vi "Generate_WayPoints_Hopping.vi"(11 "Input Cluster":T2={"Scan Rate (um/s)"=15.0, "X Start"=15.0, "X End"=15.0, "Y Start"=15.0, "Y End"=15.0, " Z Start"=15.0, "HoppingDistance"=1.0, "V"=15.0, "Z End"=15.0, "Approach Rate Hopping (um/s)"=15.0, "Retract Rate (um/s)"=15.0, "V 2"=15.0, "Approach Rate (um/s)"=15.0, "RetractV (V "=15.0}) -> (0 "output cluster":T1)   [LabVIEW 2023]
uses:
  TypeDefs/WayPointCluster.ctl
  User_Vi/Settings.vi
panel:
  in  "WayPointCluster":T1
  out "Y  P":dbl
  out "X  P":dbl
  out "HoppingDistanceX":dbl
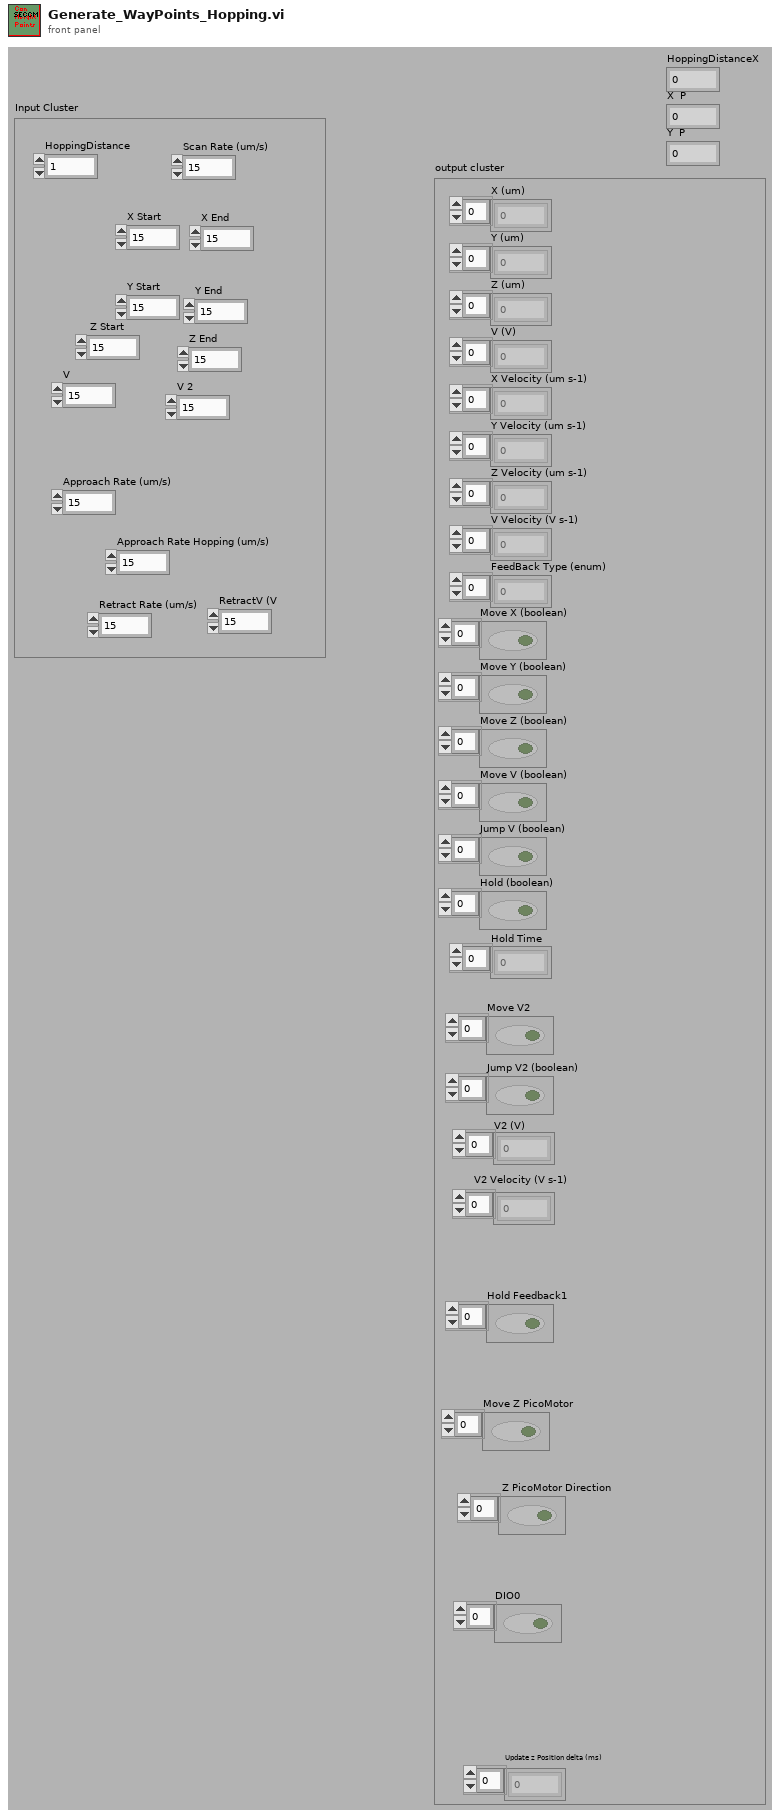
[diagram p1: front panel]
types:
  T1 = typedef "WayPointCluster.ctl" = cluster{"X (um)":dbl[], "Y (um)":dbl[], "Z (um)":dbl[], "V (V)":dbl[], "X Velocity (um s-1)":dbl[], "Y Velocity (um s-1)":dbl[], "Z Velocity (um s-1)":dbl[], "V Velocity (V s-1)":dbl[], "FeedBack Type (enum)":u16[], "Move X (boolean)":bool[], "Move Y (boolean)":bool[], "Move Z (boolean)":bool[], "Move V (boolean)":bool[], "Jump V (boolean)":bool[], "Hold (boolean)":bool[], "Hold Time":u32[], "V2 (V)":dbl[], "Move V2":bool[], "V2 Velocity (V s-1)":dbl[], "Jump V2 (boolean)":bool[], "Update z Position delta (ms)":i16[], "Hold Feedback1":bool[], "Move Z PicoMotor":bool[], " Z PicoMotor Direction":bool[], "DIO0":bool[]}
  T2 = cluster{"Scan Rate (um/s)":dbl, "X Start":dbl, "X End":dbl, "Y Start":dbl, "Y End":dbl, " Z Start":dbl, "HoppingDistance":dbl, "V":dbl, "Z End":dbl, "Approach Rate Hopping (um/s)":dbl, "Retract Rate (um/s)":dbl, "V 2":dbl, "Approach Rate (um/s)":dbl, "RetractV (V ":dbl}
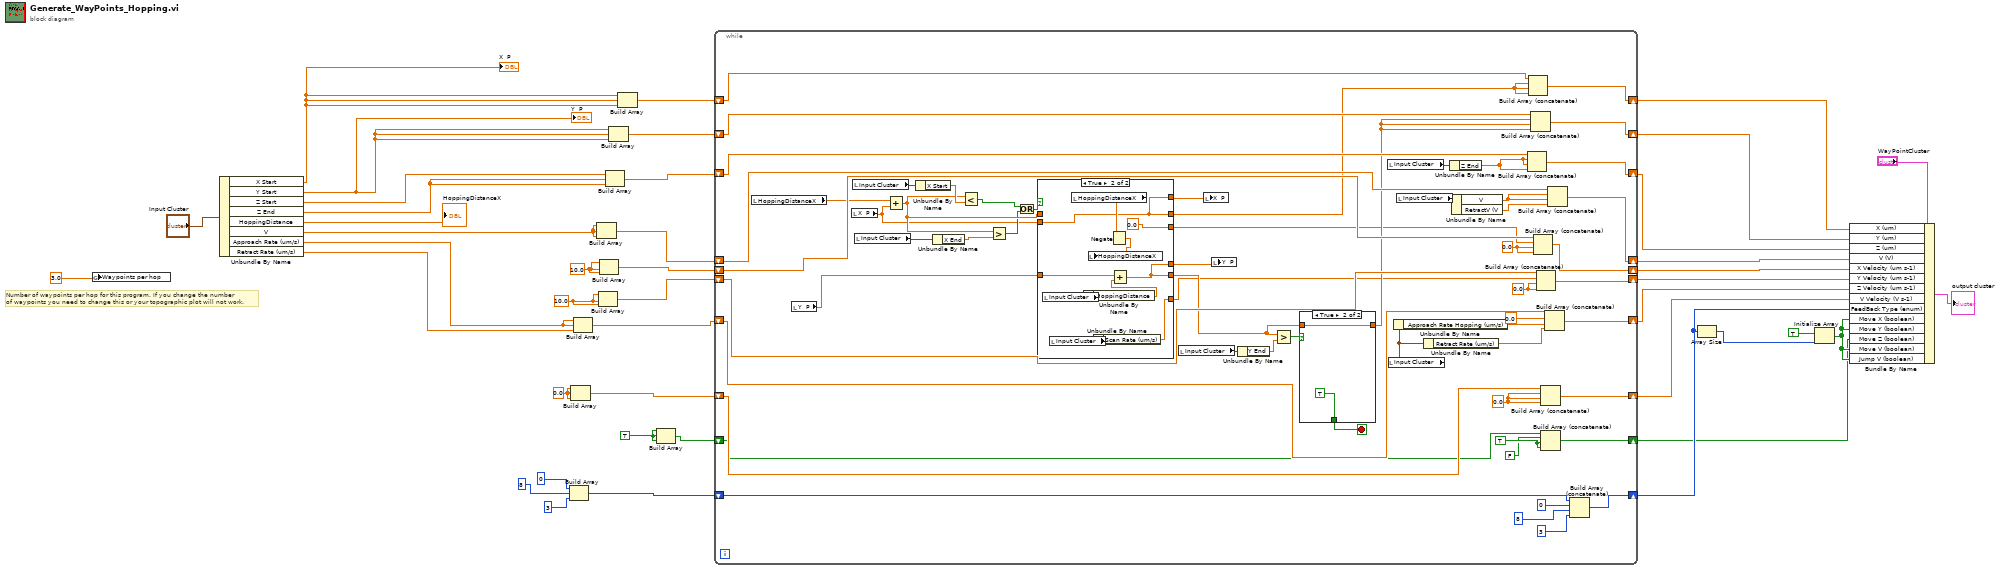
[diagram p0: block diagram]
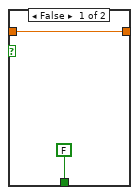
[diagram p2: hidden frame]
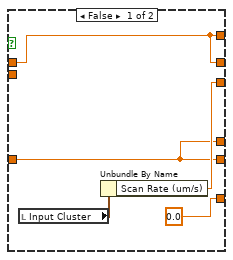
[diagram p3: hidden frame]
diagram:
  w2 = TRUE
  w12 = 10.0 ("element")
  w11 = 10.0 ("element")
  w9 = 0.0 ("element")
  # "Number of waypoints per hop for this program. If you change the number\nof waypoints you need to change this or your topographic plot will not work."
  n1 = global write "Settings.vi" "Waypoints per hop"(3.0) -> ()
  n2 = Unbundle By Name("Input Cluster") -> ("X Start"=w24:dbl, "Y Start"=w18:dbl, "Z Start"=w17:dbl, "Z End"=w14:dbl, "HoppingDistance"=→"HoppingDistanceX":dbl, "V"=w15:dbl, "Approach Rate (um/s)"=w10:dbl, "Retract Rate (um/s)"=w23:dbl)
  "X  P" <- w24
  "Y  P" <- w18
  n3 = Build Array(u16 0 ("element"), u16 8 ("element"), u16 3 ("element")) -> (w25:u16[])
  n4 = Build Array(w9, w9, w9) -> (w27:dbl[])
  n5 = Build Array(w10, w10, w23) -> (w29:dbl[])
  n6 = Build Array(w15, w15, w15) -> (w34:dbl[])
  n7 = Build Array(w11, w11, w11) -> (w31:dbl[])
  n8 = Build Array(w12, w12, w12) -> (w32:dbl[])
  n9 = Build Array(w17, w14, w14) -> (w36:dbl[])
  n10 = Build Array(w18, w18, w18) -> (w37:dbl[])
  n11 = Build Array(w24, w24, w24) -> (w39:dbl[])
  n12 = Build Array(w2, w2, w2) -> (w3:bool[])
  n13 = while {
    shift-right: [w98] -> w38
    shift-left: w39 -> [w99]
    shift-right: [w90] -> w19
    shift-left: w37 -> [w80]
    shift-right: [w89] -> w35
    shift-left: w36 -> [w97]
    shift-right: [w88] -> w33
    shift-left: w34 -> [w96]
    shift-right: [w87] -> w20
    shift-left: w32 -> [w95]
    shift-right: [w86] -> w30
    shift-left: w31 -> [w94]
    shift-right: [w85] -> w28
    shift-left: w29 -> [w93]
    shift-right: [w84] -> w26
    shift-left: w27 -> [w92]
    shift-right: [w83] -> w16
    shift-left: w25 -> [w91]
    shift-right: [w45] -> w4
    shift-left: w3 -> [w44]
    stop <- w70 stop-if-true
    w47 = TRUE
    w52 = 0.0 ("element")
    w53 = 0.0 ("element")
    w66 = 0.0 ("element")
    n14 = local read "HoppingDistanceX"() -> (w49:dbl)
    n15 = local read "Y  P"() -> (w64:dbl)
    n16 = local read "X  P"() -> (w50:dbl)
    n17 = local read "Input Cluster"() -> (w101:T2)
    n18 = local read "Input Cluster"() -> (w100:T2)
    n19 = Add(x=w49, y=w50) -> (x+y=w76:dbl)
    n20 = Unbundle By Name(w101) -> ("X Start"=w79:dbl)
    n21 = Unbundle By Name(w100) -> ("X End"=w77:dbl)
    n22 = Less?(x=w76, y=w79) -> (x < y?=w78:bool)
    n23 = Greater?(x=w76, y=w77) -> (0:w75:bool)
    n24 = Or(x=w78, y=w75) -> (x .or. y?=w74:bool)
    n25 = case shown="True" w74 {
      tunnel: w76 -> [w106 _]
      tunnel: [w106 w112] -> w63
      tunnel: w50 -> [_ w112]
      tunnel: w64 -> [w107 w113]
      tunnel: [w107 w111] -> w62
      tunnel: [w109 0.0] -> w54
      tunnel: [0.0 w114] -> w51
      tunnel: [w107 w111] -> w61
      tunnel: [w106 w112] -> w60
      frame False {
        n26 = local read "Input Cluster"() -> (w110:T2)
        n27 = Unbundle By Name(w110) -> ("Scan Rate (um/s)"=w109:dbl)
      }
      frame True {
        n28 = local read "Input Cluster"() -> (w118:T2)
        n29 = local read "Input Cluster"() -> (w116:T2)
        n30 = local read "HoppingDistanceX"() -> (w120:dbl)
        n31 = Unbundle By Name(w118) -> ("HoppingDistance"=w117:dbl)
        n32 = Unbundle By Name(w116) -> ("Scan Rate (um/s)"=w114:dbl)
        n33 = Negate(x=w120) -> (-x=w119:dbl)
        n34 = local write "HoppingDistanceX"(w119) -> ()
        n35 = Add(x=w113, y=w117) -> (x+y=w111:dbl)
      }
    }
    n36 = local read "Input Cluster"() -> (w73:T2)
    n37 = local write "X  P"(w60) -> ()
    n38 = local write "Y  P"(w61) -> ()
    n39 = Unbundle By Name(w73) -> ("Y End"=w72:dbl)
    n40 = Greater?(x=w62, y=w72) -> (0:w71:bool)
    n41 = case shown="True" w71 {
      tunnel: w62 -> [w103 w105]
      tunnel: [w103 w105] -> w69
      tunnel: [FALSE TRUE] -> w70
      frame False {
      }
      frame True {
      }
    }
    n42 = local read "Input Cluster"() -> (w82:T2)
    n43 = local read "Input Cluster"() -> (w65:T2)
    n44 = Unbundle By Name(w65) -> ("Approach Rate Hopping (um/s)"=w56:dbl)
    n45 = local read "Input Cluster"() -> (w81:T2)
    n46 = Unbundle By Name(w65) -> ("Retract Rate (um/s)"=w55:dbl)
    n47 = Unbundle By Name(w82) -> ("Z End"=w68:dbl)
    n48 = Unbundle By Name(w81) -> ("V"=w67:dbl, "RetractV (V"=w43:dbl)
    n49 = Build Array (concatenate)(w97, w68, w68, w68) -> (w89:dbl[])
    n50 = Build Array (concatenate)(w99, w63, w63, w63) -> (w98:dbl[])
    n51 = Build Array (concatenate)(w80, w69, w69, w69) -> (w90:dbl[])
    n52 = Build Array (concatenate)(w95, w54, w53, w53) -> (w87:dbl[])
    n53 = Build Array (concatenate)(w94, w51, w52, w52) -> (w86:dbl[])
    n54 = Build Array (concatenate)(w92, w66, w66, w66) -> (w84:dbl[])
    n55 = Build Array (concatenate)(w44, FALSE, w47, w47) -> (w45:bool[])
    n56 = Build Array (concatenate)(w93, 0.0 ("element"), w56, w55) -> (w85:dbl[])
    n57 = Build Array (concatenate)(w96, w67, w67, w43) -> (w88:dbl[])
    n58 = Build Array (concatenate)(w91, u16 0 ("element"), u16 8 ("element"), u16 3 ("element")) -> (w83:u16[])
  }
  n59 = Array Size(array=w16) -> (size(s)=w21:i32)
  n60 = Initialize Array(TRUE, w21) -> (w40:bool[])
  n61 = Bundle By Name(cluster="WayPointCluster", "X (um)"=w38, "Y (um)"=w19, "Z (um)"=w35, "V (V)"=w33, "X Velocity (um s-1)"=w20, "Y Velocity (um s-1)"=w30, "Z Velocity (um s-1)"=w28, "V Velocity (V s-1)"=w26, "FeedBack Type (enum)"=w16, "Move X (boolean)"=w40, "Move Y (boolean)"=w40, "Move Z (boolean)"=w4, "Move V (boolean)"=w40, "Jump V (boolean)"=w40) -> (→"output cluster":T1)
